vi "TimingSourceInitializationVI_Good.vi"(8 "error in (no error)":errorcluster, 10 "Loop Time (usec)":u32, 11 "Device Ref":T1=18446744073709551615 format="%.0x") -> (0 "error out":errorcluster, 1 "Primary Control Loop dt":i64, 2 "Actual Loop Rate (Hz)":dbl, 3 "Timing Source Name":string, 4 "Do not destroy the custom timing source":bool)   [LabVIEW 2015]
uses:
  <vilib>/NI Veristand/Custom Device API/Custom Device Item Ref.ctl
  <vilib>/NI Veristand/Custom Device API/Custom Device API.lvlib
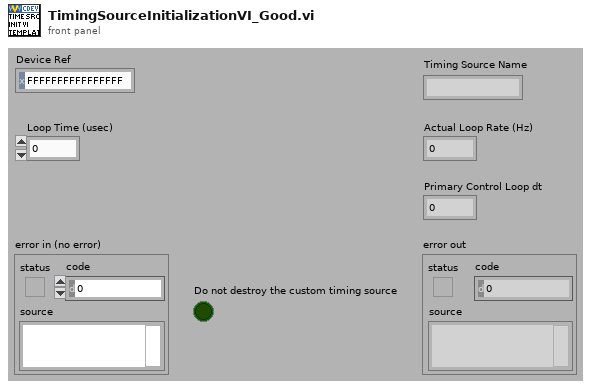
[diagram p1: front panel]
types:
  T1 = typedef "Custom Device API.lvlib/Custom Device Item Ref.ctl" = u64
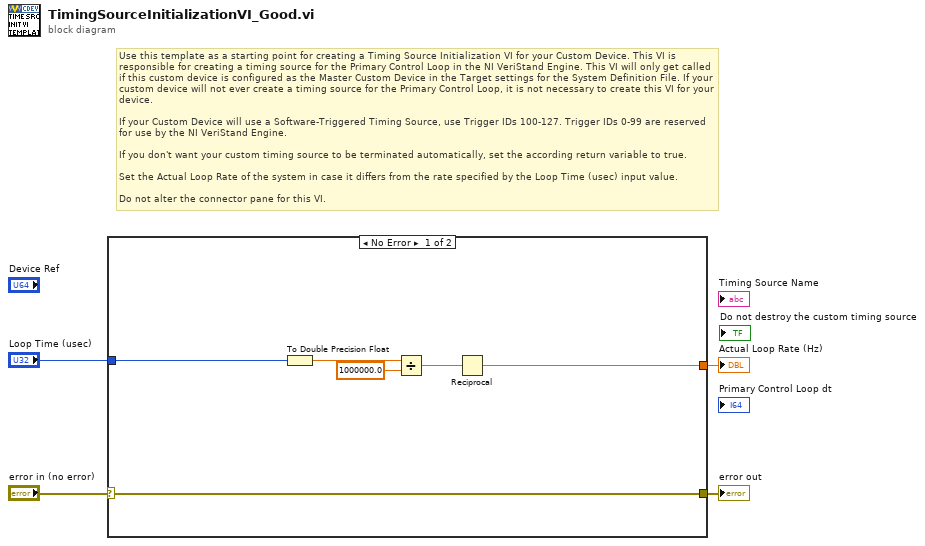
[diagram p0: block diagram]
diagram:
  # "Use this template as a starting point for creating a Timing Source Initialization VI for your Custom Device. This VI is responsible for creating a timing source for the Primary Control Loop in the NI VeriStand Engine. This VI will only get called if this custom device is configured as the Master Custom Device in the Target settings for the System Definition File. If your custom device will not ever create a timing source for the Primary Control Loop, it is not necessary to create this VI for your device.\n\nIf your Custom Device will use a Software-Triggered Timing Source, use Trigger IDs 100-127. Trigger IDs 0-99 are reserved for use by the NI VeriStand Engine.\n\nIf you don't want your custom timing source to be terminated automatically, set the according return variable to true.\n\nSet the Actual Loop Rate of the system in case it differs from the rate specified by the Loop Time (usec) input value.\n\nDo not alter the connector pane for this VI."
  n1 = case shown="No Error" "error in (no error)" {
    selector: "error in (no error)" -> [w10 w11]
    tunnel: [w10 w11] -> w4
    tunnel: "Loop Time (usec)" -> [w9 _]
    tunnel: [w5 _] -> w1
    frame No Error {
      n2 = To Double Precision Float(number=w9) -> (double precision float=w8:dbl)
      n3 = Divide(x=w8, y=1000000.0) -> (x/y=w6:dbl)
      n4 = Reciprocal(x=w6) -> (1/x=w5:dbl)
    }
    frame Error {
    }
  }
  "error out" <- w4
  "Actual Loop Rate (Hz)" <- w1
